vi "FITS - Remove Empty Table Rows.vi"(1 "Table":string[][](table)=[["0", "1"], ["10", "100"], ["20", "100"], ["30", "60"], ["40", "20"], ["50", "0"], ["", ""]]) -> (0 "Table with empty trailers removed":string[][](table)=[["0", "1"], ["10", "100"], ["20", "100"], ["30", "60"], ["40", "20"], ["50", "0"]])   [LabVIEW 2014]
doc: "Removes trailing empty rows from a table with any number of rows and columns."
panel:
  out "sizes out":i32[](array[numeric])
  out "sizes in":i32[](array[numeric])
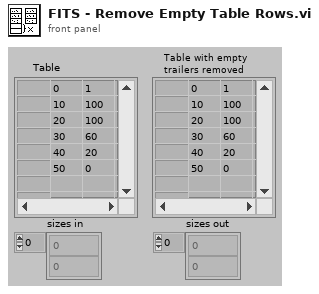
[diagram p1: front panel]
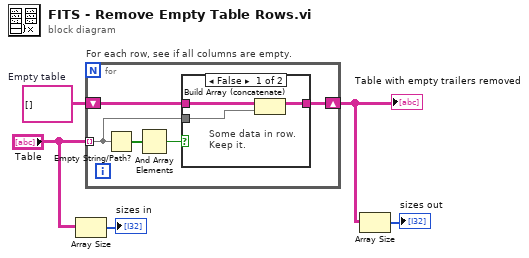
[diagram p0: block diagram]
diagram:
  w5 = string[][] []  # Empty table
  n1 = Array Size(array="Table") -> (size(s)=→"sizes in":i32[])
  n2 = for "For each row, see if all columns are empty." {
    tunnel: "Table" -> [w6] mode=indexing
    shift-right: [w7] -> w2
    shift-left: w5 -> [w8]
    n3 = Empty String/Path?(string/path=w6) -> (empty?=w10:bool[])
    n4 = And Array Elements(Boolean array=w10) -> (logical AND=w9:bool)
    n5 = case shown="False" w9 {
      tunnel: w8 -> [w13 w14]
      tunnel: [w11 w14] -> w7
      tunnel: w6 -> [w12 _]
      frame False {
        # "Some data in row.\nKeep it."
        n6 = Build Array (concatenate)(w13, w12) -> (w11:string[][])
      }
      frame True {
        # "Entire row is empty.\nIgnore it."
      }
    }
  }
  "Table with empty trailers removed" <- w2
  n7 = Array Size(array=w2) -> (size(s)=→"sizes out":i32[])
